vi "Write Database.vi"(8 "error in (no error)":errorcluster, 10 "Database":variant, 11 "Sequence Call Step Dictionary in":refnum<class "Sequence Call Step Dictionary.lvclass">) -> (0 "error out":errorcluster, 3 "Sequence Call Step Dictionary out":refnum<class "Sequence Call Step Dictionary.lvclass">)   [LabVIEW 2018, in "Sequence Call Step Dictionary.lvlib" / "Sequence Call Step Dictionary.lvclass"]
uses:
  Sequence Call Step Dictionary.lvclass
  Sequence Call Step Dictionary.lvclass/Sequence Call Step Dictionary.ctl
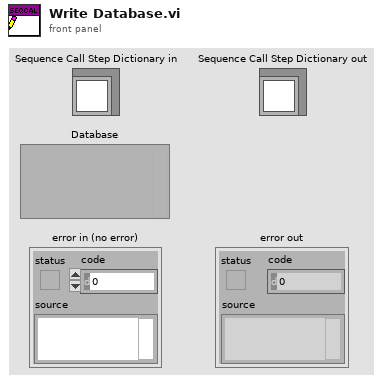
[diagram p1: front panel]
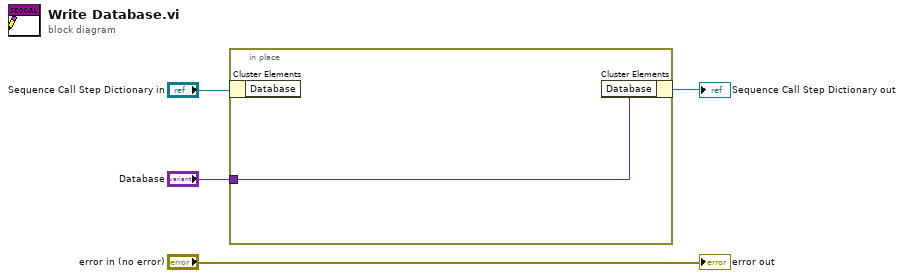
[diagram p0: block diagram]
diagram:
  n1 = in-place {
    in-place-border: "Database" -> [w5]
    n2 = in-place-cluster #1("Sequence Call Step Dictionary in") -> ()  [unwired: 1 out]
    n3 = in-place-cluster #1("Database"=w5) -> (→"Sequence Call Step Dictionary out":refnum<class "Sequence Call Step Dictionary.lvclass">)
  }
  "error out" <- "error in (no error)"
